vi "HEWH Start Stop SU Qr Index.vi"(0 "UEF Calculated Values in":T1 {"Data Indexes"."15 sec after Draw Index" format="%#.2f"; "Data Indexes"."15 sec after Draw Timestamp" format="%#.2f"; "Data Indexes"."Test Start Timestamp" format="%.2f"; "Data Indexes"."Test End Timestamp" format="%.2f"; "Data Indexes"."T0 Timestamp" format="%.2f"; "Data Indexes"."Tsf Timestamp" format="%.2f"; "Data Indexes"."Tsu0 Timestamp" format="%.2f"; "Data Indexes"."Tmax1 Timestamp" format="%.2f"; "Data Indexes"."Draw Index Timestamp" format="%#.2f"; "Data Indexes"."Non-Draw Timestamp" format="%#.2f"; "Data Indexes"."Heating Timestamp" format="%#.2f"; "Data Indexes"."Start Energy (BTU-Gas)" format="%.6f"; "Data Indexes"."Start Watt Hours" format="%.6f"; "Static Data"."V - Volume of Wh (True)" format="%.5f"; "Static Data"."T-Ambinet Nominal (°F)" format="%.5f"; "Static Data"."T-Inlet Setpoint (°F)" format="%.5f"; "Static Data"."T-Wh Setpoint (°F)" format="%.5f"; "Sampled Data"."Qe (Wh)" format="%.5f"; "Sampled Data"."Tau stby2 (hr)" format="%.5f"; "Sampled Data"."Tastby2 (°F)" format="%.5f"; "Sampled Data"."Qf (BTU)" format="%.5f"; "Sampled Data"."Qe (BTU)" format="%.5f"; "Sampled Data"."Tmax1 (°F)" format="%.5f"; "Sampled Data"."T0 (°F)" format="%.5f"; "Sampled Data"."Qr (BTU)" format="%.5f"; "Sampled Data"."T 24(°F)" format="%.5f"; "Sampled Data"."T astby(°F)" format="%.5f"; "Sampled Data"."T tstby(°F)" format="%.5f"; "Sampled Data"."T su0(°F)" format="%.5f"; "Sampled Data"."T suf(°F)" format="%.5f"; "Sampled Data"."Tau stby_1 (hr)" format="%.5f"; "Sampled Data"."Qsuf (BTU)" format="%.5f"; "Sampled Data"."Qsu0 (BTU)" format="%.5f"; "Calculated Values"."Draw Bonus Volume (gal)" format="%.6f"; "Calculated Values"."Adjustment Factor" format="%.6f"; "Calculated Values"."T*avg_del(n-1)" format="%.6f"; "Calculated Values"."T*min(n-1)" format="%.6f"; "Calculated Values"."T*avg_del(n)" format="%.6f"; "Calculated Values"."Vn" format="%.6f"; "Calculated Values"."Qdm (BTU)" format="%.6f"; "Calculated Values"."QHWD (BTU)" format="%.6f"; "Calculated Values"."QHW (BTU)" format="%.6f"; "Calculated Values"."UEF" format="%.6f"; "Calculated Values"."QHW67 (BTU)" format="%.6f"; "Calculated Values"."Qda (BTU)" format="%.6f"; "Calculated Values"."Qd (BTU)" format="%.6f"; "Calculated Values"."Q (BTU)" format="%.6f"; "Calculated Values"."UA (BTU/(hr*F))" format="%.6f"; "Calculated Values"."Qhr (BTU/hr)" format="%.6f"; "Calculated Values"."Qstby (BTU)" format="%.6f"; "Calculated Values"."nu_r" format="%.6f"; "Calculated Values"."CpUEF (BTU/(lb*F))" format="%.6f"; "Calculated Values"."rho_nu (lb/gal)" format="%.6f"; "Calculated Values"."V1- Vol (Gal)" format="%.6f"; "Calculated Values"."M cluster mass removed (lb)" format="%.6f"; "Calculated Values"."Cp theoretical (BTU/(lbm °F))" format="%.6f"; "Calculated Values"."Tin1 - Mean Inlet 1st Cluster (°F)" format="%.6f"; "Calculated Values"."Tdel1-Mean Outlet 1st Cluster(°F)" format="%.6f"; "Calculated Values"."Cp 24 (BTU/(lb*F))" format="%.6f"; "Calculated Values"."Cp standby (BTU/(lb*F))" format="%.6f"; "Calculated Values"."Cp2 (BTU/(lb*F))" format="%.6f"; "Calculated Values"."Cp1 (BTU/(lb*F))" format="%.6f"; "Calculated Values"."rho 24 (lb/gal)" format="%.6f"; "Calculated Values"."rho standby (lb/gal)" format="%.6f"; "Calculated Values"."rho 2 (lb/gal)" format="%.6f"; "Calculated Values"."Density of cold water All (lbm/gal)" format="%#.3g"; "Calculated Values"."CpHW (BTU/(lbm °F))" format="%#.3g"; "Calculated Values"."Density of hot water All (lbm/gal)" format="%#.3g"; "Calculated Values"."Mass of water All (lbm)" format="%#.3f"}, 9 "For Loop Index":i32, 11 "error in (no error)":errorcluster) -> (8 "Take5MinSample":u8, 13 "Start Index":i32, 14 "End Index":i32, 15 "error out":errorcluster)   [LabVIEW 2023]
uses:
  Type Definitions/UEF Constants.ctl
  Type Definitions/HEWH Draw Stats.ctl
  Type Definitions/HEWH FHR Draw Type.ctl
  Type Definitions/FHR Bins.ctl
  Type Definitions/HEWH Meter Type.ctl
panel:
  out "subarray 2":i32[](array[numeric])
  out "subarray":i32[](array[numeric])
  in  "Water Heater Type":string(combo)
  in  "Heat Pump (Heat Pump) 2":i32[][](array[numeric])=[[500, 4543], [14227, 17075], [24131, 26311]]
  in  "Heat Pump (Heat Pump)":i32[](array[numeric])=[2845, 3169]
  in  "Draw Index (Gas Storage)":i32[](array[numeric])=[3121, 3449]
  in  "Gas Heating Index (Gas Storage)":i32[][](array[numeric])=[[47, 1107], [1242, 1362], [1732, 1779], [3170, 3610], [14187, 14722], [15804, 16042], [16746, 16789], [17898, 18000], [18197, 18237], [22250, 22347], [22837, 22939], [23404, 23491], [23961, 24047], [24507, 25023]]
  in  "Heating Index (50 Gal Std Electric)":i32[][](array[numeric])=[[338, 744], [755, 2075], [14195, 15239], [23885, 25361]]
  in  "Draw Index (50 Gal Std Electric)":i32[](array[numeric])=[3093, 3417]
  in  "Heating Index (30 Gal Std Electric)":i32[][](array[numeric])=[[221, 1180], [2992, 3498], [13926, 14456], [16493, 16662], [17883, 17999], [22467, 22635], [24007, 24372]]
  in  "Draw Index (30 Gal Std Electric)":i32[](array[numeric])=[2841, 3165]
  out "Software Timestamp":dbl
  # "FHR"
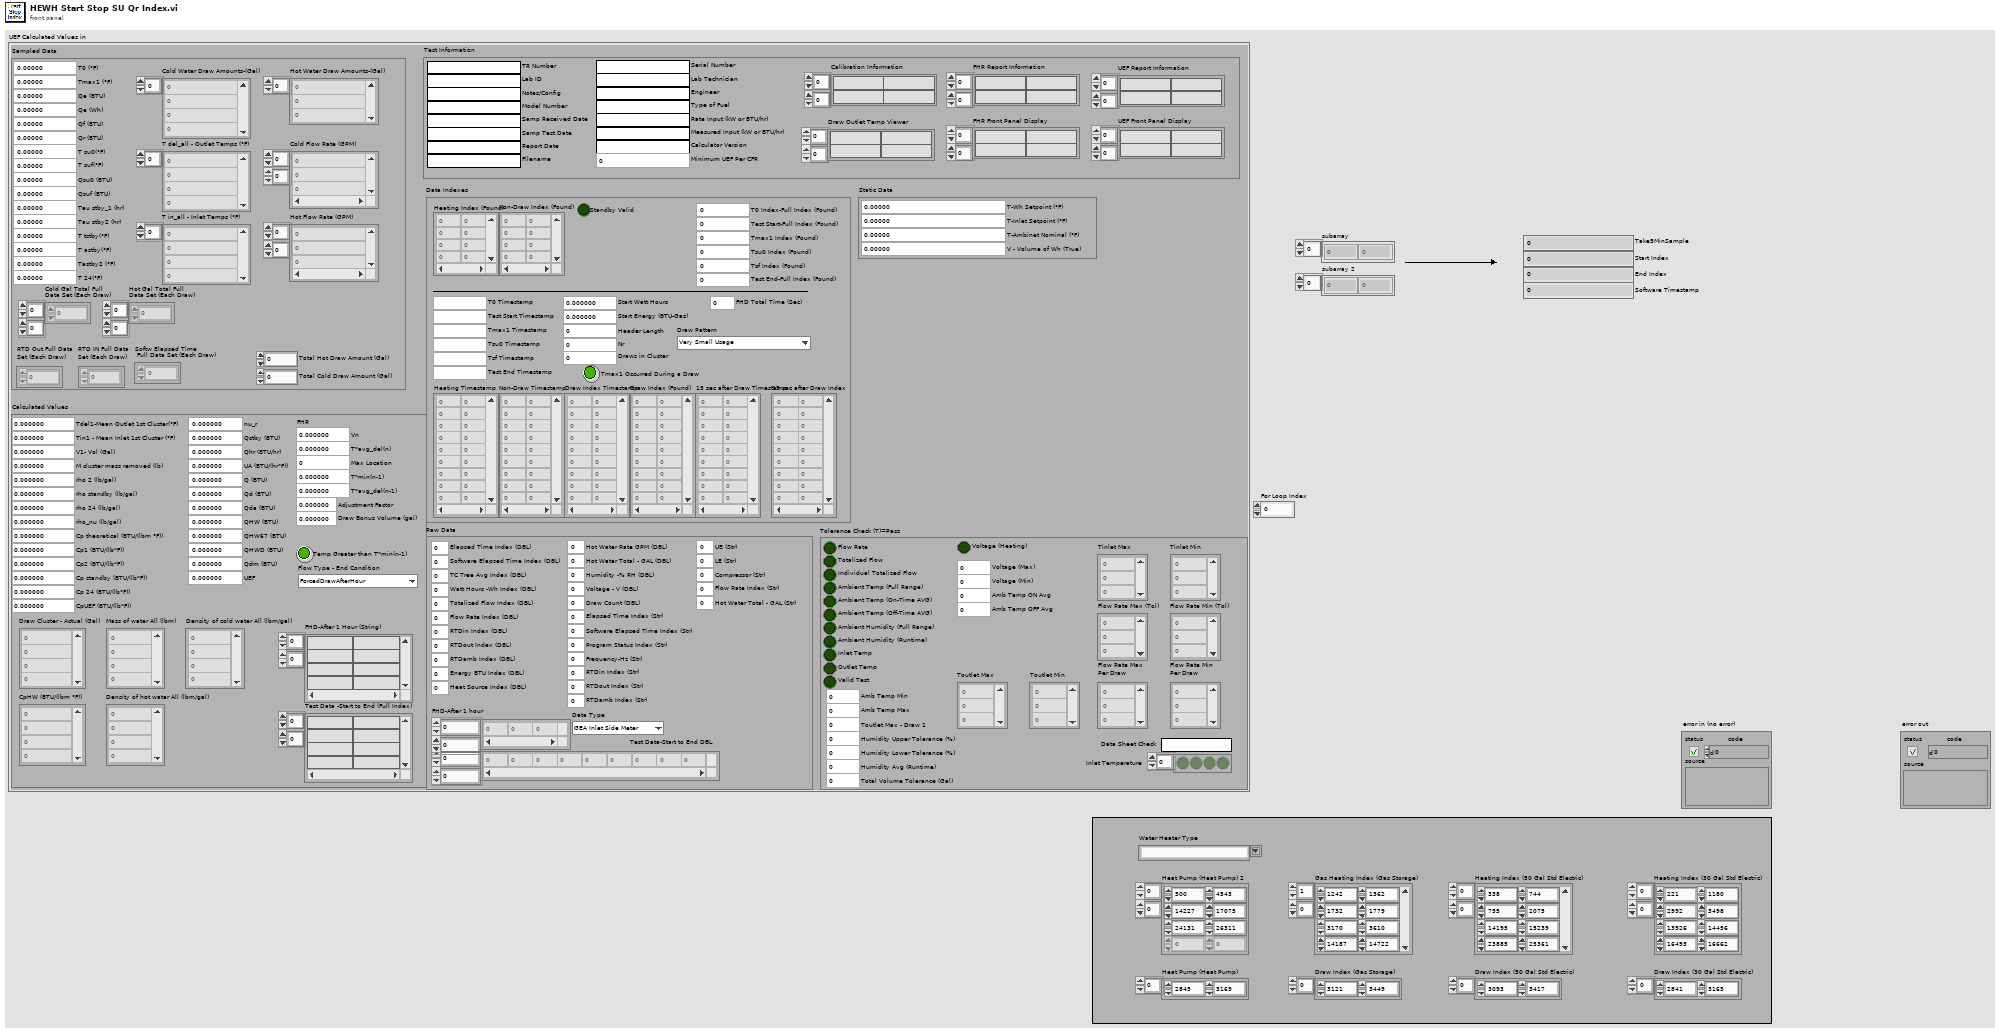
[diagram p1: front panel]
types:
  T1 = typedef "UEF Constants.ctl" = cluster{"Calculated Values":T2, "Sampled Data":cluster{"Cold Water Draw Amounts-(Gal)":dbl[], "T del_all - Outlet Temps (°F)":dbl[], "T in_all - Inlet Temps (°F)":dbl[], "Qsu0 (BTU)":dbl, "Qsuf (BTU)":dbl, "Tau stby_1 (hr)":dbl, "T suf(°F)":dbl, "T su0(°F)":dbl, "T tstby(°F)":dbl, "T astby(°F)":dbl, "T 24(°F)":dbl, "Qr (BTU)":dbl, "T0 (°F)":dbl, "Tmax1 (°F)":dbl, "Qe (BTU)":dbl, "Qf (BTU)":dbl, "Tastby2 (°F)":dbl, "RTD Out Full Data\nSet (Each Draw)":dbl[][], "RTD IN Full Data\nSet (Each Draw)":dbl[][], "Tau stby2 (hr)":dbl, "Hot Water Draw Amounts-(Gal)":dbl[], "Cold Flow Rate (GPM)":dbl[][], "Hot Flow Rate (GPM)":dbl[][], "Softw Elapsed Time\n Full Data Set (Each Draw)":dbl[][], "Cold Gal Total Full\nData Set (Each Draw)":dbl[][], "Total Hot Draw Amount (Gal) ":dbl, "Total Cold Draw Amount (Gal)":dbl, "Qe (Wh)":dbl, "Hot Gal Total Full\nData Set (Each Draw)":dbl[][]}, "Static Data":cluster{"T-Wh Setpoint (°F)":dbl, "T-Inlet Setpoint (°F)":dbl, "T-Ambinet Nominal (°F)":dbl, "V - Volume of Wh (True)":dbl}, "Data Indexes":cluster{"Test Start-Full Index (Found)":i32, "Header Length":i32, "Draw Index (Found)":i32[][], "Nr":i32, "Start Watt Hours":dbl, "Tsu0 Index (Found)":i32, "Tsf Index (Found)":i32, "Start Energy (BTU-Gas)":dbl, "Draws in Cluster":i32, "T0 Index-Full Index (Found)":i32, "Non-Draw Index (Found)":i32[][], "Tmax1 Index (Found)":i32, "Test End-Full Index (Found)":i32, "Heating Index (Found)":i32[][], "Heating Timestamp":dbl[][], "Non-Draw Timestamp":dbl[][], "Draw Index Timestamp":dbl[][], "Tmax1 Timestamp":dbl, "Tsu0 Timestamp":dbl, "Tsf Timestamp":dbl, "T0 Timestamp":dbl, "Test End Timestamp":dbl, "Test Start Timestamp":dbl, "15 sec after Draw Timestamp":dbl[][], "15 sec after Draw Index":dbl[][], "Tmax1 Occurred During a Draw":bool, "FHD Total Time (Sec)":dbl, "Draw Pattern":T4, "Standby Valid":bool}, "Raw Data":cluster{"Elapsed Time Index (DBL)":i32, "Software Elapsed Time Index (DBL)":i32, "TC Tree Avg Index (DBL)":i32, "Watt Hours -Wh Index (DBL)":i32, "Energy BTU Index (DBL)":i32, "Totalized Flow Index (DBL)":i32, "Flow Rate Index (DBL)":i32, "Program Status Index (Str)":i32, "RTDin Index (DBL)":i32, "RTDout Index (DBL)":i32, "RTDamb Index (DBL)":i32, "Test Data-Start to End DBL":dbl[][], "Data Type":T5, "Heat Source Index (DBL)":i32, "Hot Water Rate GPM (DBL)":i32, "Hot Water Total - GAL (DBL)":i32, "FHD-After 1 hour":dbl[][], "Humidity -% RH (DBL)":i32, "Voltage - V (DBL)":i32, "Draw Count (DBL)":i32, "Elapsed Time Index (Str)":i32, "Software Elapsed Time Index (Str)":i32, "Frequency-Hz (Str)":i32, "RTDin Index (Str)":i32, "RTDout Index (Str)":i32, "RTDamb Index (Str)":i32, "UE (Str)":i32, "LE (Str)":i32, "Compressor (Str)":i32, "Flow Rate Index (Str)":i32, "Hot Water Total - GAL (Str)":i32}, "Tolerance Check (T)=Pass":cluster{"Flow Rate":bool, "Totalized Flow":bool, "Ambient Temp (Full Range)":bool, "Ambient Humidity (Full Range)":bool, "Inlet Temp":bool, "Outlet Temp":bool, "Valid Test":bool, "Individual Totalized Flow":bool, "Data Sheet Check":string, "Inlet Temperature":bool[], "Tinlet Max":dbl[], "Tinlet Min":dbl[], "Flow Rate Max (Tol)":dbl[], "Flow Rate Min (Tol)":dbl[], "Amb Temp Max":dbl, "Amb Temp Min":dbl, "Toutlet Max - Draw 1":dbl, "Humidity Upper Tolerance (%)":dbl, "Total Volume Tolerance (Gal)":dbl, "Humidity Lower Tolerance (%)":dbl, "Flow Rate Max\nPer Draw":dbl[], "Flow Rate Min\nPer Draw":dbl[], "Ambient Humidity (Runtime)":bool, "Humidity Avg (Runtime)":dbl, "Ambient Temp (On-Time AVG)":bool, "Ambient Temp (Off-Time AVG)":bool, "Amb Temp OFF Avg":dbl, "Amb Temp ON Avg":dbl, "Voltage (Heating)":bool, "Voltage (Min)":dbl, "Voltage (Max)":dbl, "Toutlet Max":dbl[], "Toutlet Min":dbl[]}, "Test Information":cluster{"TR Number":string, "Lab ID":string, "Notes/Config":string, "Model Number":string, "Serial Number":string, "Lab Technician":string, "Engineer":string, "Type of Fuel":string, "Samp Received Date":string, "Samp Test Date":string, "Report Date":string, "Rate Input (kW or BTU/hr)":string, "Measured Input (kW or BTU/hr)":string, "Filename":string, "Calibration Information":string[][], "Calculator Version":string, "Minimum UEF Per CFR":dbl, "UEF Report Information":string[][], "FHR Report Information":string[][], "FHR Front Panel Display":string[][], "UEF Front Panel Display":string[][], "Draw Outlet Temp Viewer":string[][]}}
  T2 = typedef "HEWH Draw Stats.ctl" = cluster{"Draw Cluster - Actual (Gal)":dbl[], "Mass of water All (lbm)":dbl[], "Density of hot water All (lbm/gal)":dbl[], "CpHW (BTU/(lbm °F))":dbl[], "rho 2 (lb/gal)":dbl, "rho standby (lb/gal)":dbl, "rho 24 (lb/gal)":dbl, "Cp1 (BTU/(lb*F))":dbl, "Cp2 (BTU/(lb*F))":dbl, "Cp standby (BTU/(lb*F))":dbl, "Cp 24 (BTU/(lb*F))":dbl, "nu_r":dbl, "Qstby (BTU)":dbl, "Qhr (BTU/hr)":dbl, "UA (BTU/(hr*F))":dbl, "Q (BTU)":dbl, "Qd (BTU)":dbl, "Qda (BTU)":dbl, "QHW67 (BTU)":dbl, "UEF":dbl, "Tdel1-Mean Outlet 1st Cluster(°F)":dbl, "Tin1 - Mean Inlet 1st Cluster (°F)":dbl, "Cp theoretical (BTU/(lbm °F))":dbl, "M cluster mass removed (lb)":dbl, "V1- Vol (Gal)":dbl, "Test Data -Start to End (Full Index)":string[][], "rho_nu (lb/gal)":dbl, "Density of cold water All (lbm/gal)":dbl[], "CpUEF (BTU/(lb*F))":dbl, "QHW (BTU)":dbl, "QHWD (BTU)":dbl, "Qdm (BTU)":dbl, "FHD-After 1 Hour (String)":string[][], "Vn":dbl, "T*avg_del(n)":dbl, "Max Location":i32, "T*min(n-1)":dbl, "T*avg_del(n-1)":dbl, "Temp Greater than T*min(n-1)":bool, "Adjustment Factor":dbl, "Draw Bonus Volume (gal)":dbl, "Flow Type - End Condition":T3}
  T3 = typedef "HEWH FHR Draw Type.ctl" = enum16{"ForcedDrawAfterHour", "HeatingCutoffBeforeHour"}
  T4 = typedef "FHR Bins.ctl" = enum16{"Very Small Usage", "Low Usage", "Medium Usage", "High Usage", "Undefined"}
  T5 = typedef "HEWH Meter Type.ctl" = enum16{"GEA Inlet Side Meter", "GEA Outlet Side Meter", "CSA Inlet Side Meter"}
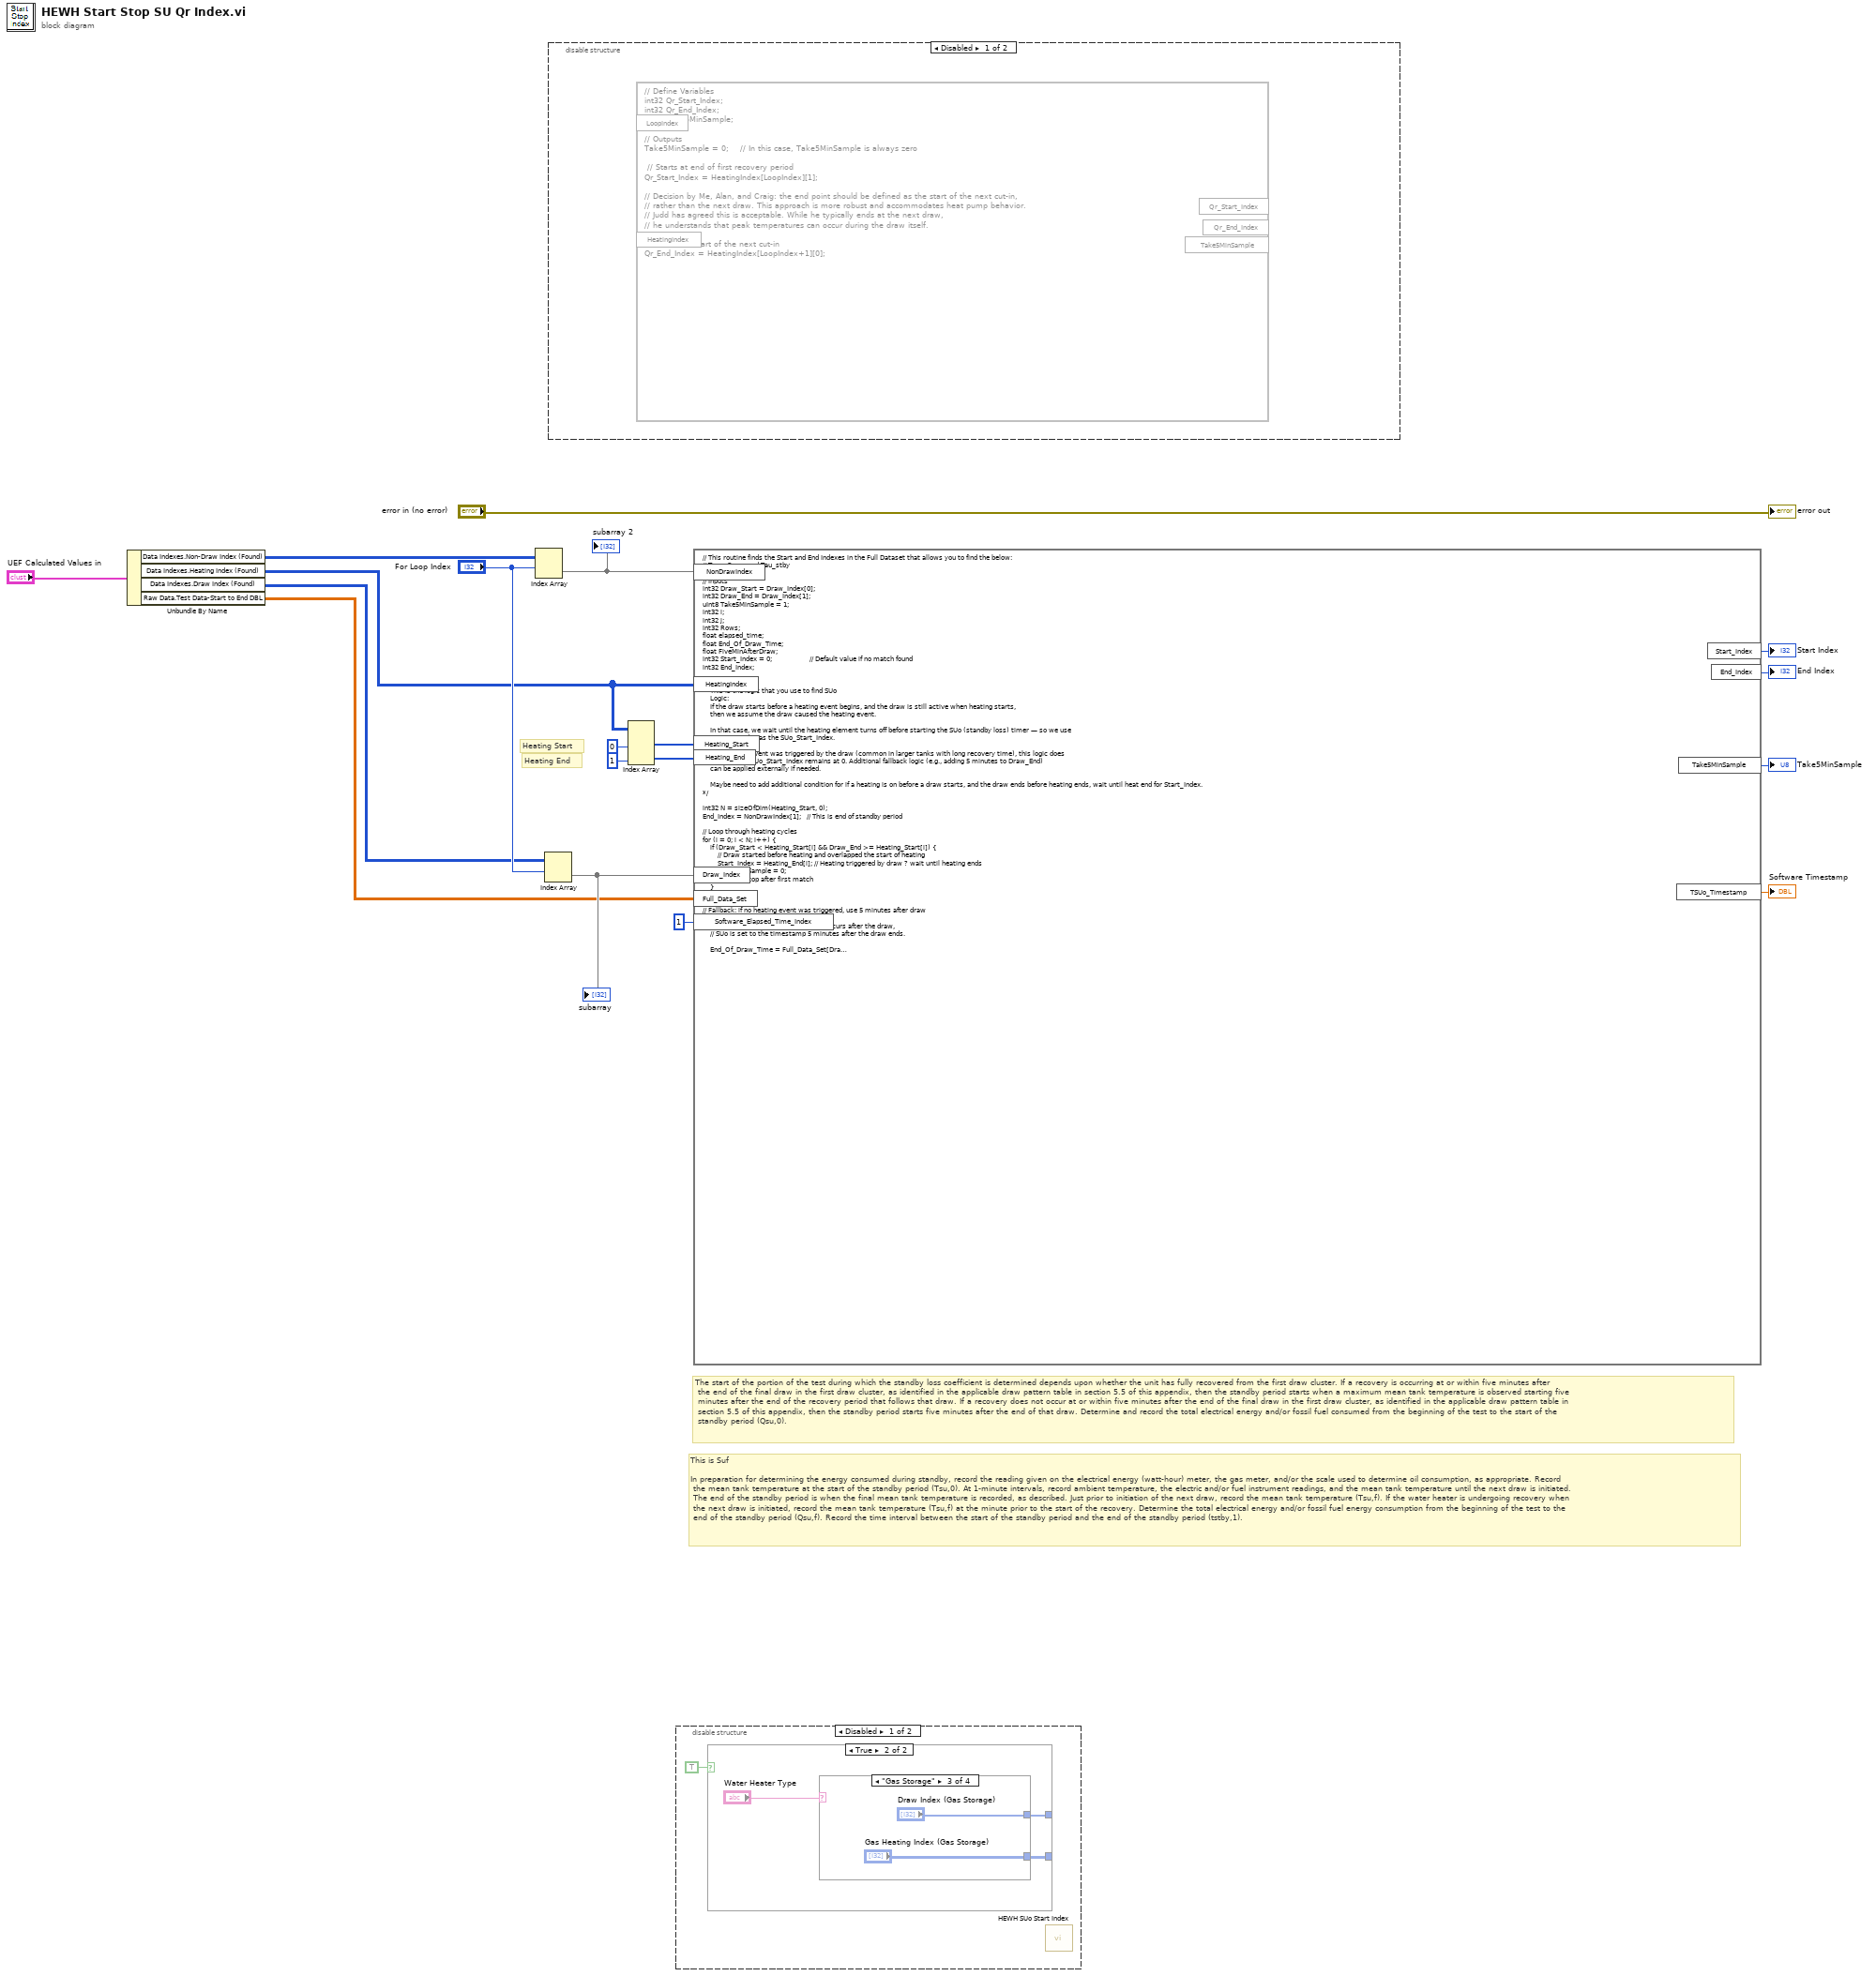
[diagram p0: block diagram]
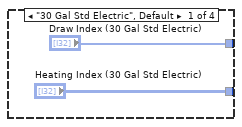
[diagram p4: hidden frame]
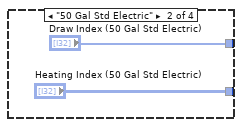
[diagram p5: hidden frame]
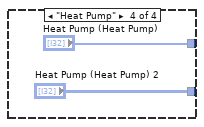
[diagram p6: hidden frame]
diagram:
  # "This is Suf\n\nIn preparation for determining the energy consumed during standby, record the reading given on the electrical energy (watt-hour) meter, the gas meter, and/or the scale used to determine oil consumption, as appropriate. Record\n the mean tank temperature at the start of the standby period (Tsu,0). At 1-minute intervals, record ambient temperature, the electric and/or fuel instrument readings, and the mean tank temperature until the next draw is initiated.\n The end of the standby period is when the final mean tank temperature is recorded, as described. Just prior to initiation of the next draw, record the mean tank temperature (Tsu,f). If the water heater is undergoing recovery when\n the next draw is initiated, record the mean tank temperature (Tsu,f) at the minute prior to the start of the recovery. Determine the total electrical energy and/or fossil fuel energy consumption from the beginning of the test to the\n end of the standby period (Qsu,f). Record the time interval between the start of the standby period and the end of the standby period (tstby,1)."
  # "The start of the portion of the test during which the standby loss coefficient is determined depends upon whether the unit has fully recovered from the first draw cluster. If a recovery is occurring at or within five minutes after\n the end of the final draw in the first draw cluster, as identified in the applicable draw pattern table in section 5.5 of this appendix, then the standby period starts when a maximum mean tank temperature is observed starting five\n minutes after the end of the recovery period that follows that draw. If a recovery does not occur at or within five minutes after the end of the final draw in the first draw cluster, as identified in the applicable draw pattern table in\n section 5.5 of this appendix, then the standby period starts five minutes after the end of that draw. Determine and record the total electrical energy and/or fossil fuel consumed from the beginning of the test to the start of the\n standby period (Qsu,0)."
  # "Heating End"
  # "Heating Start"
  n1 = Unbundle By Name("UEF Calculated Values in") -> ("Data Indexes.Non-Draw Index (Found)"=w4:i32[][], "Data Indexes.Heating Index (Found)"=w3:i32[][], "Data Indexes.Draw Index (Found)"=w2:i32[][], "Raw Data.Test Data-Start to End DBL"=w1:dbl[][])
  n2 = Index Array(array=w4, index (row)="For Loop Index") -> (element=w8:i32[])  [unwired: 1 in]
  "subarray 2" <- w8
  n3 = Index Array(array=w2, index (row)="For Loop Index") -> (element=w7:i32[])  [unwired: 1 in]
  "subarray" <- w7
  n4 = disable-structure shown="Disabled" {
    frame Disabled {
      n5 = formula code="// Define Variables\nint32 Qr_Start_Index;\nint32 Qr_End_Index;\nuInt8 Take5MinSample;\n\n// Outputs\nTake5MinSample = 0;    // In this case, Take5MinSample is always zero\n\n // Starts at end of first recovery period\nQr_Start_Index = HeatingIndex[LoopIndex][1];  \n\n// Decision by Me, Alan, and Craig: the end point should be defined as the start of the next cut-in,\n// rather than the next draw. This approach is more robust and accommodates heat pump behavior.\n// Judd has agreed this is acceptable. While he typically ends at the next draw,\n// he understands that peak temperatures can occur during the draw itself.\n\n// This is the start of the next cut-in\nQr_End_Index = HeatingIndex[LoopIndex+1][0];"() -> ()  [unwired: 2 in, 3 out]
    }
    frame Enabled {
    }
  }
  n6 = Index Array "Index Array"(array=w3, index (col) #1=0 ("disabled index (col)"), index (col) #2=1 ("index (col)")) -> (element #1=w13:i32[], element #2=w14:i32[])  [unwired: 2 in]
  n7 = disable-structure shown="Disabled" {
    frame Disabled {
      n8 = case shown="True" TRUE {
        tunnel: [_ w21] -> _
        tunnel: [_ w20] -> _
        frame False {
        }
        frame True {
          n9 = case shown="\"Gas Storage\"" "Water Heater Type" {
            tunnel: ["Heating Index (30 Gal Std Electric)" "Heating Index (50 Gal Std Electric)" "Gas Heating Index (Gas Storage)" "Heat Pump (Heat Pump) 2"] -> w21
            tunnel: ["Draw Index (30 Gal Std Electric)" "Draw Index (50 Gal Std Electric)" "Draw Index (Gas Storage)" "Heat Pump (Heat Pump)"] -> w20
            frame "30 Gal Std Electric", Default {
            }
            frame "50 Gal Std Electric" {
            }
            frame "Gas Storage" {
            }
            frame "Heat Pump" {
            }
          }
        }
      }
      n10 = call "HEWH SUo Start Index.vi"() -> ()  [unwired: 9 in, 3 out]
    }
    frame Enabled {
    }
  }
  n11 = formula code="// This routine finds the Start and End Indexes in the Full Dataset that allows you to find the below:\n// Tsuo, Qsuo, and Tau_stby\n\n// Inputs\nint32 Draw_Start = Draw_Index[0];\nint32 Draw_End = Draw_Index[1];\nuInt8 Take5MinSample = 1;\nint32 i;\nint32 j;\nint32 Rows;\nfloat elapsed_time;\nfloat End_Of_Draw_Time;\nfloat FiveMinAfterDraw;\nint32 Start_Index = 0;                    // Default value if no match found\nint32 End_Index;\n\n/*\n    This is the logic that you use to find SUo    \n    Logic:\n    If the draw starts before a heating event begins, and the draw is still active when heating starts,\n    then we assume the draw caused the heating event.\n\n    In that case, we wait until the heating element turns off before starting the SUo (standby loss) timer — so we use\n    Heating_End[i] as the SUo_Start_Index.\n\n    If no heating event was triggered by the draw (common in larger tanks with long recovery time), this logic does\n    nothing, and SUo_Start_Index remains at 0. Additional fallback logic (e.g., adding 5 minutes to Draw_End)\n    can be applied externally if needed.\n\n    Maybe need to add additional condition for if a heating is on before a draw starts, and the draw ends before heating ends, wait until heat end for Start_Index.\n*/\n\nint32 N = sizeOfDim(Heating_Start, 0);\nEnd_Index = NonDrawIndex[1];   // This is end of standby period\n\n// Loop through heating cycles\nfor (i = 0; i < N; i++) {\n    if (Draw_Start < Heating_Start[i] && Draw_End >= Heating_Start[i]) {\n        // Draw started before heating and overlapped the start of heating\n        Start_Index = Heating_End[i]; // Heating triggered by draw ? wait until heating ends\n        Take5MinSample = 0;\n        break; // Stop after first match\n    }\n}\n\n// Fallback: if no heating event was triggered, use 5 minutes after draw\nif (Take5MinSample == 1) {\n    // When no heating element activity occurs after the draw,\n    // SUo is set to the timestamp 5 minutes after the draw ends.\n\n    End_Of_Draw_Time = Full_Data_Set[Draw_End][Software_Elapsed_Time_Index];\n    FiveMinAfterDraw = End_Of_Draw_Time + 300;\n    \n    Rows = sizeOfDim(Full_Data_Set, 0);\n\n    for (j = Draw_End; j < Rows; j++) {\n        elapsed_time = Full_Data_Set[j][Software_Elapsed_Time_Index];\n\n        if (elapsed_time >= FiveMinAfterDraw) {\n            Start_Index = j;\n            TSUo_Timestamp = Full_Data_Set[j][Software_Elapsed_Time_Index]; // Store the timestamp at that index // Optional: save timestamp for reporting\n            break;\n        }\n    }\n}"("Heating_Start"=w13, "Draw_Index"=w7, "Heating_End"=w14, "Full_Data_Set"=w1, "Software_Elapsed_Time_Index"=1 ("disabled index (col)"), "NonDrawIndex"=w8, "HeatingIndex"=w3) -> ("Start_Index"=→"Start Index":i32, "Take5MinSample"=→"Take5MinSample":u8, "TSUo_Timestamp"=→"Software Timestamp":dbl, "End_Index"=→"End Index":i32)
  "error out" <- "error in (no error)"
